vi "Sequence-Start tracking.vi"   [LabVIEW 2020]
uses:
  Global Variables/gl_UI Ctrl Refs.vi
types:
  T1 = enum8{"Enabled", "Disabled", "Disabled and Grayed Out"}
  T2 = typedef "UI ctrl refs cluster.ctl" = cluster{"Top level VI path":path, "Top level VI ref":refnum<vi>, "User menu ref":refnum<k9>, "Sub Panel control":refnum<vi>, "Imaging Param Tab":refnum<vi>, "Occurrence-Start drivers":refnum<k4>, "Occurrence-Speed logging initialised":refnum<k4>, "Occurrence-XYZ stage initialised":refnum<k4>, "Exit button":refnum<vi>, "Status ind":refnum<vi>, "Set as origin":refnum<vi>, "Speed Logging":refnum<vi>, "Time Lapse":refnum<vi>, "Live Imaging":refnum<vi>, "AOL Z Stack":refnum<vi>, "Motor Z Stack":refnum<vi>, "Funct Acq button":refnum<vi>, "Hard Shutter":refnum<vi>, "Virtual Shutter":refnum<vi>, "Laser Power":refnum<vi>, "AOL Mode":refnum<vi>, "Frame Size":refnum<vi>, "Field of View":refnum<vi>, "Dwell Time":refnum<vi>, "Zoom":refnum<vi>, "AOL Z":refnum<vi>, "Objective":refnum<vi>, "Axis":refnum<vi>, "Paths & Names":refnum<vi>, "Experiment folder path (ind.)":refnum<vi>, "Last State (Ind.)":refnum<vi>, "Averages":refnum<vi>, "Angle (degrees)":refnum<vi>, "X centre":refnum<vi>, "Y centre":refnum<vi>, "Plane Mode":refnum<vi>, "# Planes":refnum<vi>, "Z Start":refnum<vi>, "Z Stop":refnum<vi>, "Z Step":refnum<vi>, "PMT 1":refnum<vi>, "PMT 2":refnum<vi>, "Stage XYZ Position":refnum<vi>, "Pockels@Z Start":refnum<vi>, "Pockels@Z Stop":refnum<vi>, "Obtain Z Start":refnum<vi>, "Obtain Z Stop":refnum<vi>, "Live stim.trig.period":refnum<vi>, "Live stim.trig.enable":refnum<vi>, "Movement Correction":refnum<vi>, "Load Reference Image":refnum<vi>, "XY Stage Move":refnum<vi>, "MovCor Cluster":refnum<vi>, "RefDAQParam":refnum<vi>, "Funct. Acq. Pockels Modulation":refnum<vi>, "Ref Laser Power":refnum<vi>, "Enable Video Recording":refnum<vi>, "Video Record-Live Imaging":refnum<vi>, "Video Record-Funct acq":refnum<vi>, "Reference Source":refnum<vi>, "AOL Z-stack Chirps Ready (ind)":refnum<vi>, "Target time between mov.cor. ref triggers (ms)":refnum<vi>, "Funct. Acq. Ref frame save":refnum<vi>, "Tracking button":refnum<vi>, "Show ref plots window":refnum<vi>, "Center freq ind (nm)":refnum<vi>, "Pickup mode (ind)":refnum<vi>, "Logging queue (ind)":refnum<vi>, "Back aperture power (ind.)":refnum<vi>, "Power after objective (ind.)":refnum<vi>, "Switch user":refnum<vi>, "Ls1 Conn. Status":refnum<vi>, "Ls1Tuning Status":refnum<vi>, "Ls1 Faults":refnum<vi>, "Ls1 Connection":refnum<vi>, "Ls1 Mode":refnum<vi>, "Ls1 POWER [mW]":refnum<vi>, "Ls1Shutter":refnum<vi>, "Ls1 Wavelength":refnum<vi>, "Ls1 Note":refnum<vi>, "Ls1 Confirm Wav":refnum<vi>, "Ls1 PreChrp Prism1":refnum<vi>, "Ls1 PreChrp Prism2":refnum<vi>, "Ls1 wav top Ind":refnum<vi>, "Ls1 power top Ind":refnum<vi>, "Ls1 Pump peak Hold":refnum<vi>, "Ls1 Status Ind":refnum<vi>, "Ls1 wav cancel":refnum<vi>, "Experiment Type":refnum<vi>, "Biology Information":refnum<vi>, "Camera recording status":refnum<vi>}
  T3 = typedef "test_fpga_control.ctl" = cluster{"x_offset_host":fxp<+/-,16,8>, "y_offset_host":fxp<+/-,16,8>, "use host offset":bool, "Set_Ref_Centroid":bool, "OldChirpCode":bool, "use array of offsets":bool, "x_offset_host array":fxp<+/-,16,8>[], "y_offset_host array ":fxp<+/-,16,8>[], "use host offset Z":bool, "swap Z":bool, "z_offset_host ":fxp<+/-,16,8>}
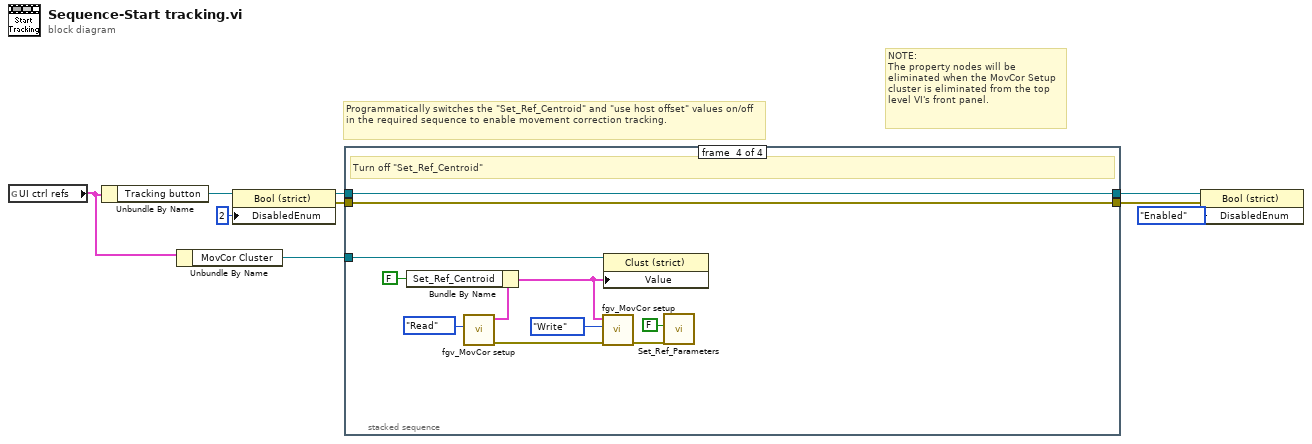
[diagram p0: block diagram]
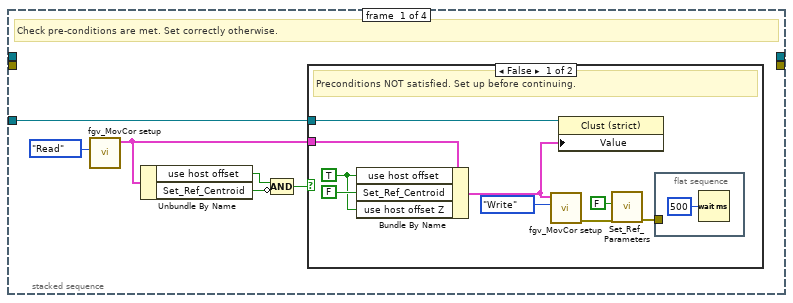
[diagram p2: hidden frame]
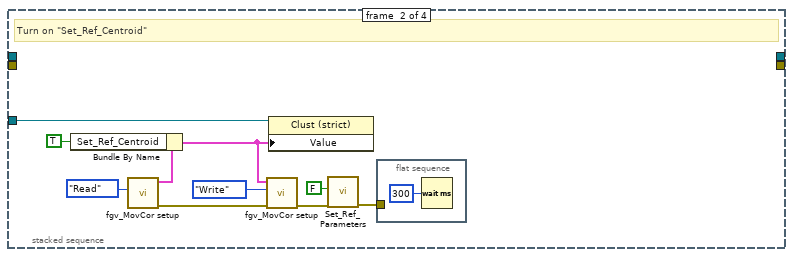
[diagram p4: hidden frame]
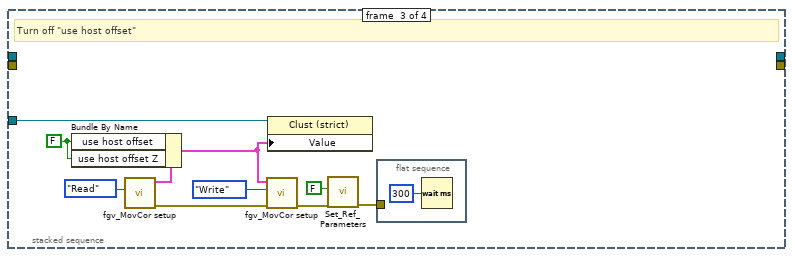
[diagram p5: hidden frame]
diagram:
  # "NOTE:\nThe property nodes will be eliminated when the MovCor Setup cluster is eliminated from the top level VI's front panel."
  # "Programmatically switches the \"Set_Ref_Centroid\" and \"use host offset\" values on/off in the required sequence to enable movement correction tracking."
  n1 = global read "gl_UI Ctrl Refs.vi" "UI ctrl refs"() -> (w2:T2)
  n2 = Unbundle By Name(w2) -> ("Tracking button"=w3:refnum<vi>)
  n3 = Unbundle By Name(w2) -> ("MovCor Cluster"=w9:refnum<vi>)
  n4 = property on="Property Node" class="Bool (strict)"(reference=w3, "DisabledEnum"=2) -> (reference out=w6:refnum<vi>, error out=w7:errorcluster)  [unwired: 1 in]
  n5 = stacked-sequence {
    tunnel: w9 -> [w10 w28 w40 w52]
    tunnel: w7 -> [_ _ _ w48]
    tunnel: [_ _ _ w49] -> w5
    tunnel: w6 -> [_ _ _ w49]
    tunnel: [_ _ _ w48] -> w4
    frame #0 {
      # "Check pre-conditions are met. Set correctly otherwise."
      n6 = call "fgv_MovCor setup.vi"("Status"=enum16{"Initialize", "Write", "Read"}."Read") -> ("MovCor Cluster"=w11:T3)  [unwired: 9 in, 1 out]
      n7 = Unbundle By Name(w11) -> ("use host offset"=w15:bool, "Set_Ref_Centroid"=w14:bool)
      n8 = Compound Arithmetic op=AND(w15, invert w14) -> (w13:bool)
      n9 = case shown="False" w13 {
        tunnel: w11 -> [w23 _]
        tunnel: w10 -> [w17 _]
        frame False {
          w16 = TRUE ("use host offset")
          # "Preconditions NOT satisfied. Set up before continuing."
          n10 = Bundle By Name(cluster=w23, "use host offset"=w16, "Set_Ref_Centroid"=FALSE, "use host offset Z"=w16) -> (w18:T3)
          n11 = call "fgv_MovCor setup.vi"("Status"=enum16{"Initialize", "Write", "Read"}."Write", "MovCor Cluster"=w18) -> ("error out"=w20:errorcluster)  [unwired: 8 in, 1 out]
          n12 = property class="Clust (strict)"(reference=w17, "Value"=w18) -> ()  [unwired: 1 in, 2 out]
          n13 = call "Set_Ref_Parameters.vi"("error in"=w20, "use_increment_halfrate"=FALSE) -> ("error out"=w19:errorcluster)  [unwired: 7 in, 2 out]
          n14 = flat-sequence {
            tunnel: w19 -> [_]
            frame #0 {
              n15 = Wait (ms)(milliseconds to wait=u32 500 ("millisecond multiple")) -> ()  [unwired: 1 out]
            }
          }
        }
        frame True {
          # "Preconditions satisfied to allow continuing"
        }
      }
    }
    frame #1 {
      # "Turn on \"Set_Ref_Centroid\""
      n16 = call "fgv_MovCor setup.vi"("Status"=enum16{"Initialize", "Write", "Read"}."Read") -> ("error out"=w26:errorcluster, "MovCor Cluster"=w29:T3)  [unwired: 9 in]
      n17 = Bundle By Name(cluster=w29, "Set_Ref_Centroid"=TRUE) -> (w27:T3)
      n18 = call "fgv_MovCor setup.vi"("error in (no error)"=w26, "Status"=enum16{"Initialize", "Write", "Read"}."Write", "MovCor Cluster"=w27) -> ("error out"=w32:errorcluster)  [unwired: 7 in, 1 out]
      n19 = property class="Clust (strict)"(reference=w28, "Value"=w27) -> ()  [unwired: 1 in, 2 out]
      n20 = call "Set_Ref_Parameters.vi"("error in"=w32, "use_increment_halfrate"=FALSE) -> ("error out"=w35:errorcluster)  [unwired: 7 in, 2 out]
      n21 = flat-sequence {
        tunnel: w35 -> [_]
        frame #0 {
          n22 = Wait (ms)(milliseconds to wait=u32 300 ("millisecond multiple")) -> ()  [unwired: 1 out]
        }
      }
    }
    frame #2 {
      w37 = FALSE ("Set_Ref_Centroid")
      # "Turn off \"use host offset\""
      n23 = call "fgv_MovCor setup.vi"("Status"=enum16{"Initialize", "Write", "Read"}."Read") -> ("error out"=w38:errorcluster, "MovCor Cluster"=w41:T3)  [unwired: 9 in]
      n24 = Bundle By Name(cluster=w41, "use host offset"=w37, "use host offset Z"=w37) -> (w39:T3)
      n25 = call "fgv_MovCor setup.vi"("error in (no error)"=w38, "Status"=enum16{"Initialize", "Write", "Read"}."Write", "MovCor Cluster"=w39) -> ("error out"=w43:errorcluster)  [unwired: 7 in, 1 out]
      n26 = property class="Clust (strict)"(reference=w40, "Value"=w39) -> ()  [unwired: 1 in, 2 out]
      n27 = call "Set_Ref_Parameters.vi"("error in"=w43, "use_increment_halfrate"=FALSE) -> ("error out"=w46:errorcluster)  [unwired: 7 in, 2 out]
      n28 = flat-sequence {
        tunnel: w46 -> [_]
        frame #0 {
          n29 = Wait (ms)(milliseconds to wait=u32 300 ("millisecond multiple")) -> ()  [unwired: 1 out]
        }
      }
    }
    frame #3 {
      # "Turn off \"Set_Ref_Centroid\""
      n30 = call "fgv_MovCor setup.vi"("Status"=enum16{"Initialize", "Write", "Read"}."Read") -> ("error out"=w50:errorcluster, "MovCor Cluster"=w53:T3)  [unwired: 9 in]
      n31 = Bundle By Name(cluster=w53, "Set_Ref_Centroid"=FALSE) -> (w51:T3)
      n32 = call "fgv_MovCor setup.vi"("error in (no error)"=w50, "Status"=enum16{"Initialize", "Write", "Read"}."Write", "MovCor Cluster"=w51) -> ("error out"=w56:errorcluster)  [unwired: 7 in, 1 out]
      n33 = property class="Clust (strict)"(reference=w52, "Value"=w51) -> ()  [unwired: 1 in, 2 out]
      n34 = call "Set_Ref_Parameters.vi"("error in"=w56, "use_increment_halfrate"=FALSE) -> ()  [unwired: 7 in, 3 out]
    }
  }
  n35 = property on="Property Node" class="Bool (strict)"(reference=w5, error in=w4, "DisabledEnum"=T1."Enabled" ("Disabled")) -> ()  [unwired: 2 out]
